vi "Get Panel from SubPanel.vi"(7 "Panel Type (Panel)":refnum<class "Panel.lvclass">, 8 "error in (no error)":errorcluster, 10 "SubPanel":refnum<vi>, 11 "Manager in":refnum<class "Manager.lvclass">) -> (0 "error out":errorcluster, 2 "Panel":refnum<class "Panel.lvclass">, 3 "Manager out":refnum<class "Manager.lvclass">)   [LabVIEW 2020, in "OOPanel.lvlib" / "Manager.lvclass"]
uses:
  Manager.lvclass
  Panel/Panel.lvclass
  Manager.lvclass/Manager.ctl
  <vilib>/Utility/error.llb/Error Cluster From Error Code.vi
  <vilib>/ErrorRing/Error Ring.xnode
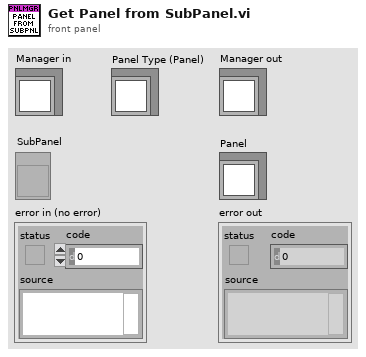
[diagram p1: front panel]
types:
  T1 = typedef "OOPanel.lvlib/Manager.lvclass/Ref Data.ctl" = cluster{"SubPanel Map":T2, "Panels":refnum<class "Panel.lvclass">[]}
  T2 = typedef "OOPanel.lvlib/Manager.lvclass/SubPanel Map.ctl" = cluster{"SubPanels":refnum<vi>[], "Panels":refnum<class "Panel.lvclass">[]}
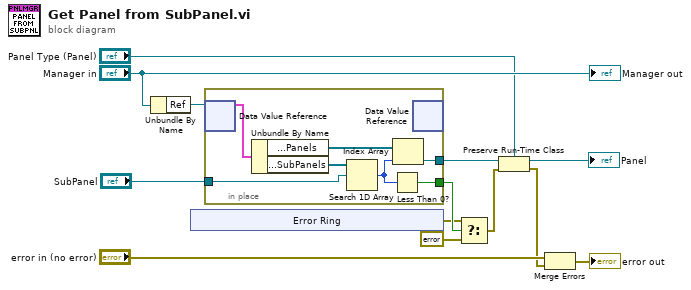
[diagram p0: block diagram]
diagram:
  n1 = Unbundle By Name("Manager in") -> ("Ref"=w12:refnum<data-value>)
  n2 = xnode "Error Ring"() -> ("error out"=w5:errorcluster)
  n3 = in-place {
    in-place-border: "SubPanel" -> [w18]
    in-place-border: [w16] -> w9
    in-place-border: [w14] -> w6
    n4 = in-place-dvr #1(w12) -> (w20:T1)  [unwired: 1 out]
    n5 = Unbundle By Name(w20) -> ("SubPanel Map.Panels"=w17:refnum<class "Panel.lvclass">[], "SubPanel Map.SubPanels"=w19:refnum<vi>[])
    n6 = Search 1D Array(1D array=w19, element=w18) -> (index of element=w15:i32)  [unwired: 1 in]
    n7 = Less Than 0?(x=w15) -> (x < 0?=w14:bool)
    n8 = Index Array(array=w17, index=w15) -> (element=w16:refnum<class "Panel.lvclass">)
    n9 = in-place-dvr #1() -> ()  [unwired: 1 in, 2 out]
  }
  n10 = Select(t=w5, s=w6, f=errorcluster {"status"=FALSE, "code"=0, "source"=""}) -> (s? t:f=w3:errorcluster)
  n11 = Preserve Run-Time Class(object in=w9, error in=w3, 2:"Panel Type (Panel)") -> (object out=→"Panel":refnum<class "Panel.lvclass">, error out=w1:errorcluster)
  n12 = Merge Errors("error in (no error)", w1) -> (→"error out":errorcluster)
  "Manager out" <- "Manager in"
